vi "Switch Configuration - Move Channels between ListBoxes.vi"(8 "error in (no error)":errorcluster, 9 "ListBox Origin In":i32[](array[numeric]), 10 "ListBox Origin Ref In":refnum<vi>, 11 "ListBox Destiny Ref In":refnum<vi>) -> (0 "error out":errorcluster, 1 "ListBox Out":i32[](array[numeric]), 2 "ListBox Origin Ref Out":refnum<vi>, 3 "ListBox Destiny Ref Out":refnum<vi>, 4 "Destiny Item Names":string[](array[string]), 6 "Origin Item Names":string[](array[string]))   [LabVIEW 2015, in "DMM-SWITCH-ScanList System Explorer.lvlib"]
doc: "This VI is called when the Add Channels or Remove Channels buttons are pressed. Copies the selected channels (ListBox Origin In Array) from Origin ListBox to Destiny ListBox, sorts the remaining channels in Destiny ListBox, and deletes the selected channels from Origin ListBox."
uses:
  DMM-SWITCH-ScanList System Explorer.lvlib
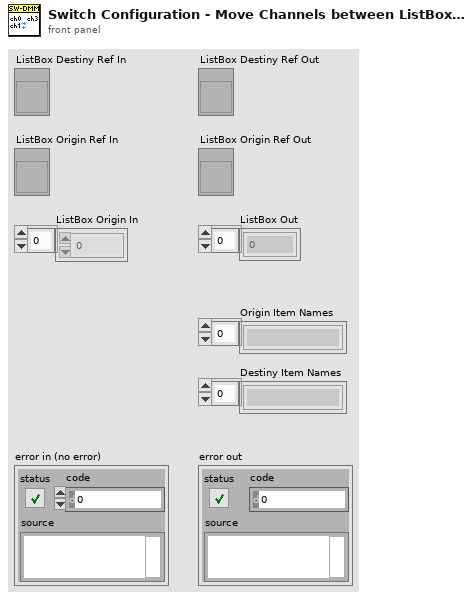
[diagram p1: front panel]
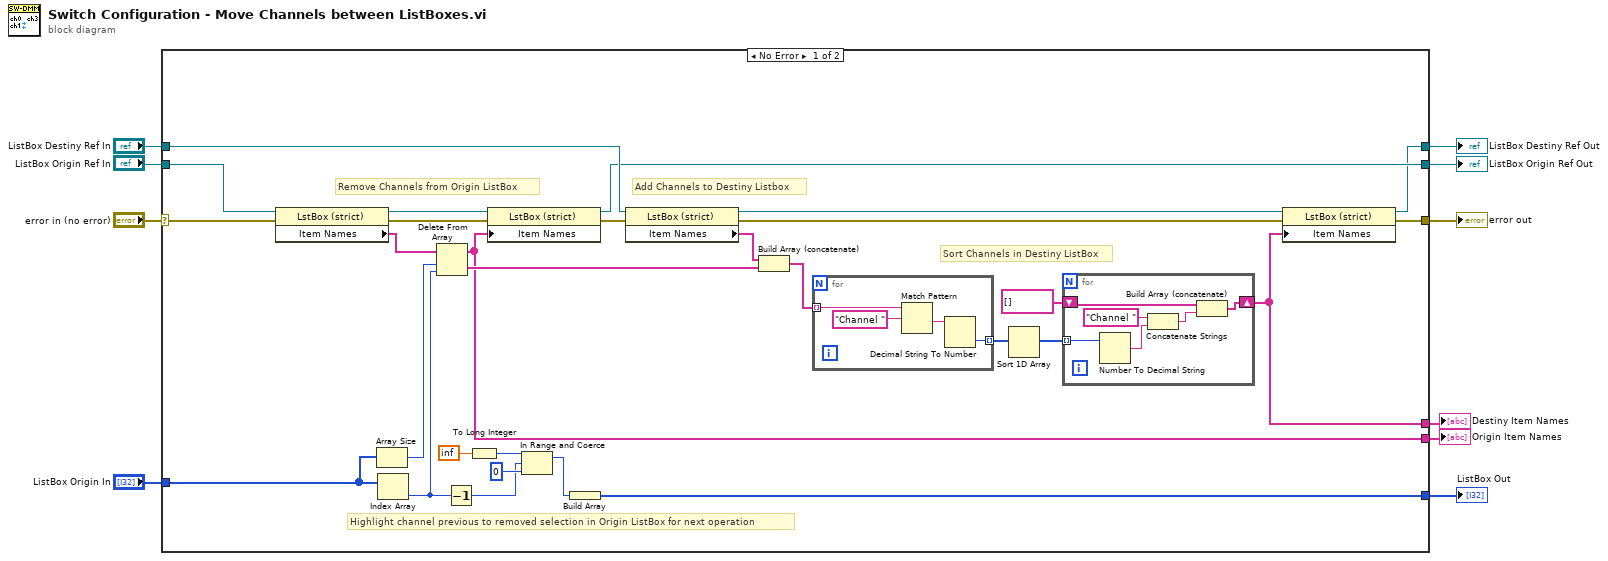
[diagram p0: block diagram]
diagram:
  n1 = case shown="No Error" "error in (no error)" {
    selector: "error in (no error)" -> [w30 w53]
    tunnel: [w21 w52] -> w10
    tunnel: [w23 w53] -> w9
    tunnel: "ListBox Destiny Ref In" -> [w34 w52]
    tunnel: "ListBox Origin Ref In" -> [w31 w51]
    tunnel: [w29 w51] -> w5
    tunnel: "ListBox Origin In" -> [w20 w50]
    tunnel: [w19 w50] -> w3
    tunnel: [w12 _] -> w2
    tunnel: [w11 _] -> w1
    frame No Error {
      # "Highlight channel previous to removed selection in Origin ListBox for next operation"
      # "Sort Channels in Destiny ListBox"
      # "Add Channels to Destiny Listbox"
      # "Remove Channels from Origin ListBox"
      n2 = property class="LstBox (strict)"(reference=w31, error in=w30) -> (reference out=w32:refnum<vi>, error out=w33:errorcluster, "Item Names"=w36:string[])
      n3 = Array Size(array=w20) -> (size(s)=w15:i32)
      n4 = Index Array(array=w20) -> (element=w39:i32)  [unwired: 1 in]
      n5 = Delete From Array(array=w36, length=w15, index=w39) -> (deleted portion=w38:string[], array with subset deleted=w11:string[])
      n6 = Decrement(x=w39) -> (x-1=w17:i32)
      n7 = To Long Integer(number=inf) -> (32bit integer=w14:i32)
      n8 = property class="LstBox (strict)"(reference=w32, error in=w33, "Item Names"=w11) -> (reference out=w29:refnum<vi>, error out=w37:errorcluster)
      n9 = In Range and Coerce(upper limit=w14, x=w17, lower limit=0) -> (coerced(x)=w16:i32)  [unwired: 1 out]
      n10 = Build Array(w16) -> (w19:i32[])
      n11 = property class="LstBox (strict)"(reference=w34, error in=w37) -> (reference out=w22:refnum<vi>, error out=w25:errorcluster, "Item Names"=w35:string[])
      n12 = Build Array (concatenate)(w35, w38) -> (w24:string[])
      n13 = for {
        tunnel: w24 -> [w48] mode=indexing
        tunnel: [w46] -> w28 mode=indexing
        n14 = Match Pattern(string=w48, regular expression="Channel ") -> (after substring=w47:string)  [unwired: 1 in, 3 out]
        n15 = Decimal String To Number(string=w47) -> (number=w46:i32)  [unwired: 2 in, 1 out]
      }
      n16 = Sort 1D Array(array=w28) -> (sorted array=w27:i32[])
      n17 = for {
        tunnel: w27 -> [w45] mode=indexing
        shift-right: [w40] -> w12
        shift-left: string[] [] ("array w/ subset deleted") -> [w44]
        n18 = Number To Decimal String(number=w45) -> (decimal integer string=w41:string)  [unwired: 1 in]
        n19 = Concatenate Strings("Channel " ("string"), w41) -> (w43:string)
        n20 = Build Array (concatenate)(w44, w43) -> (w40:string[])
      }
      n21 = property class="LstBox (strict)"(reference=w22, error in=w25, "Item Names"=w12) -> (reference out=w21:refnum<vi>, error out=w23:errorcluster)
    }
    frame Error {
    }
  }
  "ListBox Destiny Ref Out" <- w10
  "error out" <- w9
  "ListBox Origin Ref Out" <- w5
  "ListBox Out" <- w3
  "Destiny Item Names" <- w2
  "Origin Item Names" <- w1
